vi "Read Message.vi"(8 "error in (no error)":errorcluster, 11 "Arduino Detector in":refnum<class "Arduino Detector.lvclass">) -> (0 "error out":errorcluster, 2 "Message":string, 3 "Arduino Detector out":refnum<class "Arduino Detector.lvclass">)   [LabVIEW 2019, in "Arduino Detector.lvclass"]
uses:
  Arduino Detector.lvclass
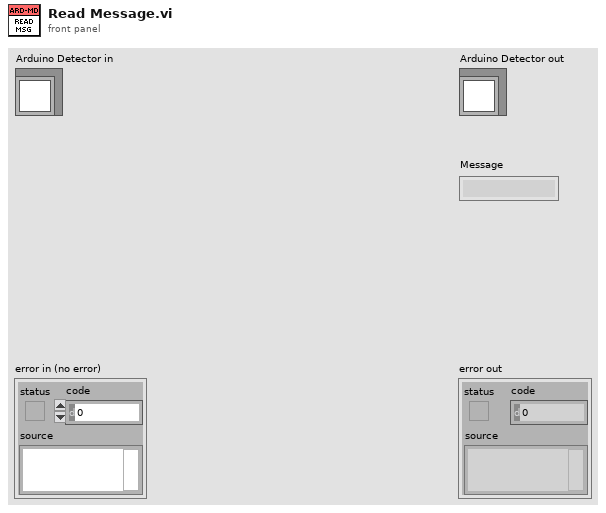
[diagram p1: front panel]
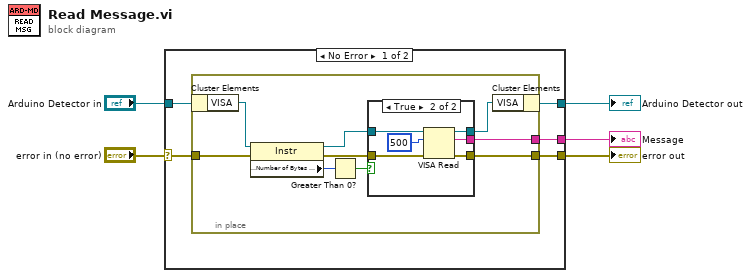
[diagram p0: block diagram]
diagram:
  n1 = case shown="No Error" "error in (no error)" {
    selector: "error in (no error)" -> [w8 w29]
    tunnel: "Arduino Detector in" -> [w10 w28]
    tunnel: [w9 w28] -> w4
    tunnel: [w7 w29] -> w2
    tunnel: [w6 _] -> w1
    frame No Error {
      n2 = in-place {
        in-place-border: w8 -> [w13]
        in-place-border: [w18] -> w7
        in-place-border: [w17] -> w6
        n3 = in-place-cluster #1(w10) -> ("VISA"=w16:refnum<visa-resource-name>)
        n4 = property class="Instr"(reference=w16, error in=w13) -> (reference out=w15:refnum<visa-resource-name>, error out=w14:errorcluster, "Serial Settings:Number of Bytes at Serial Port"=w12:u32)
        n5 = Greater Than 0?(x=w12) -> (x > 0?=w11:bool)
        n6 = case shown="True" w11 {
          tunnel: [w21 w27] -> w19
          tunnel: [w20 w26] -> w18
          tunnel: [_ w25] -> w17
          tunnel: w15 -> [w21 w23]
          tunnel: w14 -> [w20 w22]
          frame False {
          }
          frame True {
            n7 = VISA Read(VISA resource name=w23, byte count=u32 500, error in (no error)=w22) -> (VISA resource name out=w27:refnum<visa-resource-name>, read buffer=w25:string, error out=w26:errorcluster)  [unwired: 1 out]
          }
        }
        n8 = in-place-cluster #1("VISA"=w19) -> (w9:refnum<class "Arduino Detector.lvclass">)
      }
    }
    frame Error {
    }
  }
  "error out" <- w2
  "Arduino Detector out" <- w4
  "Message" <- w1
